vi "Turn Set and Get.vi"(8 "error in (no error)":errorcluster, 11 "Manejador de Turnos in":refnum<class "Manejador de Turnos.lvclass">) -> (0 "error out":errorcluster, 3 "Manejador de Turnos out":refnum<class "Manejador de Turnos.lvclass">)   [LabVIEW 2021, in "Manejador de Turnos.lvlib" / "Manejador de Turnos.lvclass"]
uses:
  Manejador de Turnos.lvclass
  Manejador de Turnos.lvclass/Manejador de Turnos.ctl
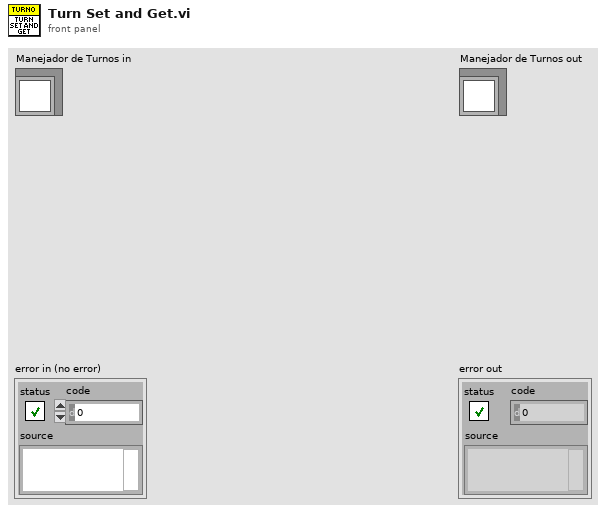
[diagram p1: front panel]
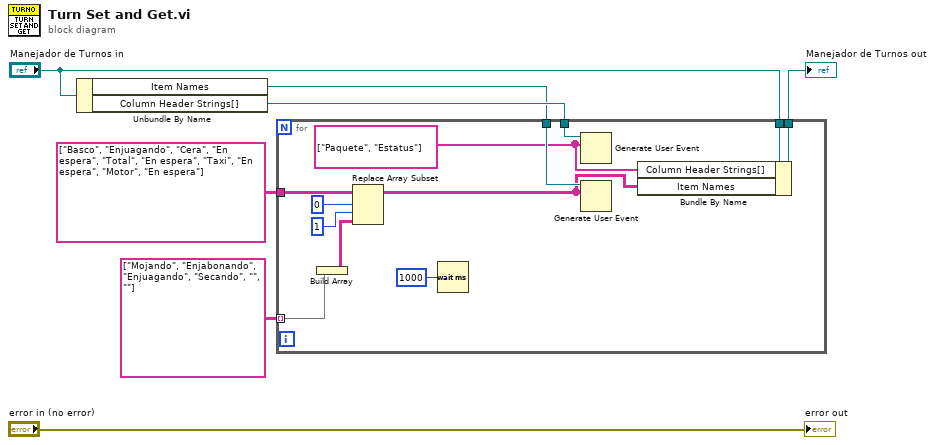
[diagram p0: block diagram]
diagram:
  n1 = Unbundle By Name("Manejador de Turnos in") -> ("Item Names"=w3:refnum<user-event>, "Column Header Strings[]"=w4:refnum<user-event>)
  n2 = for {
    tunnel: string[][] [["Basco", "Enjuagando"], ["Cera", "En espera"], ["Total", "En espera"], ["Taxi", "En espera"], ["Motor", "En espera"]] ("Item Names") -> [w18]
    tunnel: string[][] [["Mojando"], ["Enjabonando"], ["Enjuagando"], ["Secando"], [""], [""]] ("Item Names") -> [w15] mode=indexing
    tunnel: w4 -> [w13]
    tunnel: w3 -> [w12]
    tunnel: "Manejador de Turnos in" -> [w11]
    tunnel: [w10] -> w1
    w9 = string[] ["Paquete", "Estatus"] ("Row Header Strings[]")
    n3 = Build Array(w15) -> (w14:string[][])
    n4 = Replace Array Subset(array=w18, new element=w14, index (row)=0 ("disabled index (row)"), index (col)=1 ("disabled index (row)")) -> (w8:string[][])
    n5 = Wait (ms)(milliseconds to wait=u32 1000) -> ()  [unwired: 1 out]
    n6 = Generate User Event(user event=w13, event data cluster=w9) -> ()  [unwired: 2 in, 2 out]
    n7 = Generate User Event(user event=w12, event data cluster=w8) -> ()  [unwired: 2 in, 2 out]
    n8 = Bundle By Name(cluster=w11, "Column Header Strings[]"=w9, "Item Names"=w8) -> (w10:refnum<class "Manejador de Turnos.lvclass">)
  }
  "Manejador de Turnos out" <- w1
  "error out" <- "error in (no error)"
